vi "cost.vi"(8 "error in (no error)":errorcluster, 11 "CondimentDecorator in":refnum<class "CondimentDecorator.lvclass">) -> (0 "error out":errorcluster, 2 "Cost":dbl, 3 "CondimentDecorator out":refnum<class "CondimentDecorator.lvclass">)   [LabVIEW 2013, in "CondimentDecorator.lvclass"]
uses:
  CondimentDecorator.lvclass
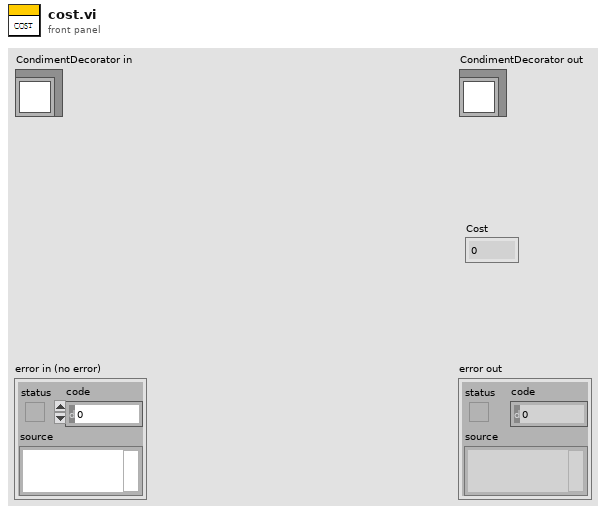
[diagram p1: front panel]
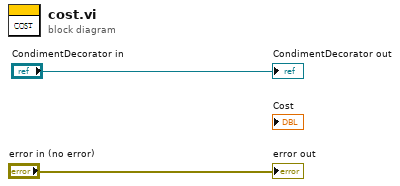
[diagram p0: block diagram]
diagram:
  "error out" <- "error in (no error)"
  "CondimentDecorator out" <- "CondimentDecorator in"
